vi "Grab and Bayer Decoding.vi"() -> ()   [LabVIEW 2011]
doc: "The Grab and Bayer Decoding VI acquires images continuously and displays the images in an image control using high-level acquisition VIs. This VI also demonstrates decoding bayer encoded patterns from the camera. A grab is appropriate for high-speed applications in which you need to process only one image at a time."
uses:
  <vilib>/vision/driver/NI_Vision_Acquisition_Software.lvlib
  resource/objmgr/imaqdx.rc
panel:
  in  "Camera Name":refnum<k21> caption="IMAQdx Session"
  in  "Bayer Parameters":T1 {"Blue Gain" scale=0.0..3.99; "Green Gain" scale=0.0..3.99; "Red Gain" scale=0.0..3.99; "Bayer Pattern" items=["None", "GB", "GR", "BG", "RG", "Use hardware value"]}
  out "Buffer Number":u32
  out "Image":T2(plugin-control)
  out "Frame Rate":dbl(knob) scale=0.0..100.0
  in  "Stop":bool
  # "Overview: Demonstrates how to modify the Bayer Parameters while acquiring a continuous acquisition.\nRequirements: Vision Acquisition Software, camera that outputs 8-bit or 16-bit Bayer images.\nInstructions: \n1. Select the Camera Name\n2. Run the VI\n3. Select the Bayer Pattern.\n4. Adjust the red, green, blue gains."
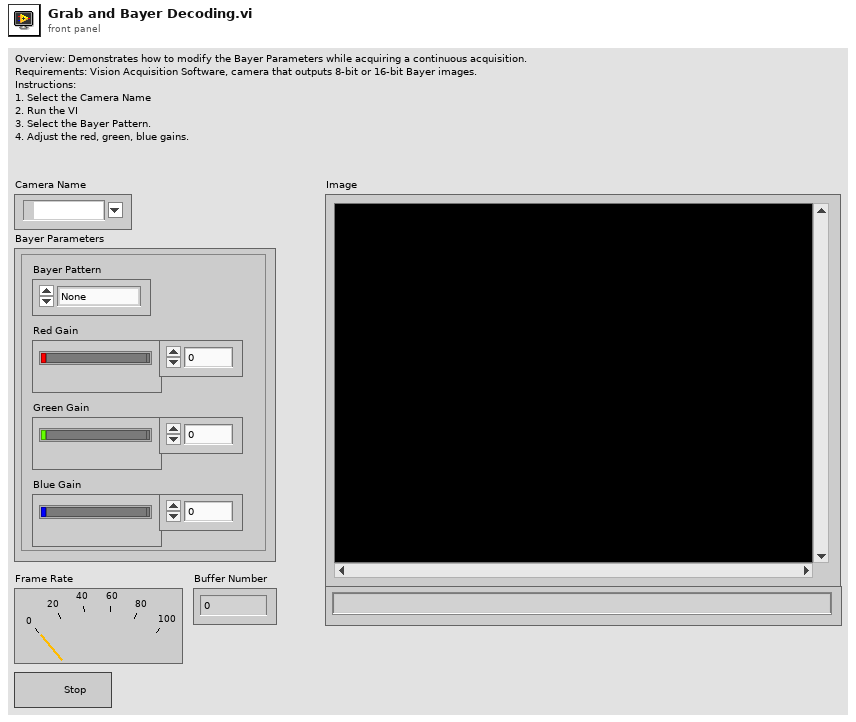
[diagram p1: front panel]
types:
  T1 = cluster{"Bayer Pattern":u32, "Red Gain":dbl, "Green Gain":dbl, "Blue Gain":dbl}
  T2 = typedef "IMAQ Image.ctl" = refnum<image>
  T3 = typedef "IMAQdx.ctl" = refnum<k21>
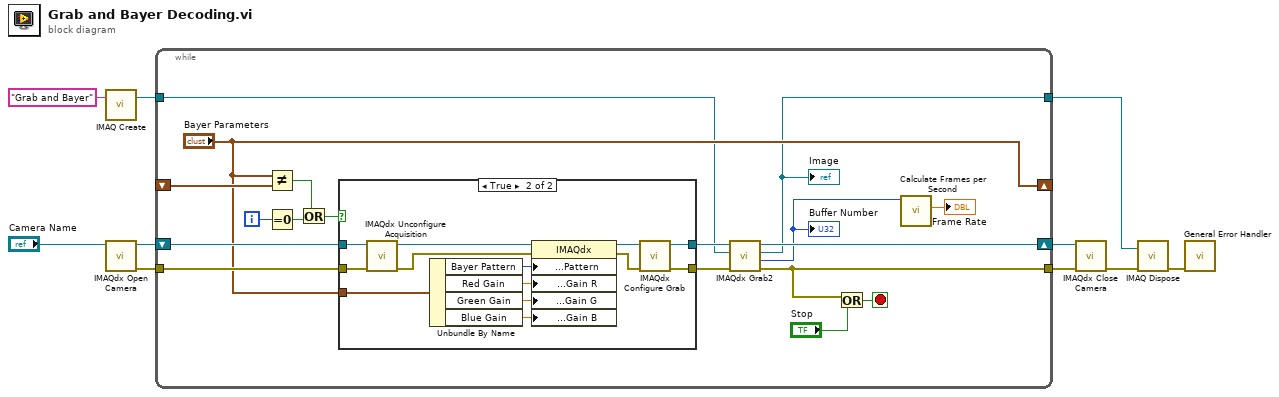
[diagram p0: block diagram]
diagram:
  n1 = call "IMAQ Create"("Image Name"="Grab and Bayer") -> ("New Image"=w10:T2)  [unwired: 3 in, 2 out]
  n2 = call <vilib>:"IMAQdx Open Camera.vi"("Session In"="Camera Name") -> ("error out"=w6:errorcluster, "Session Out"=w7:T3)  [unwired: 2 in, 7 out]
  n3 = while {
    tunnel: [w13] -> w8
    tunnel: w10 -> [w12]
    shift-right: ["Bayer Parameters"] -> _
    shift-left: _ -> [w21]
    tunnel: w6 -> [w22]
    shift-right: [w26] -> w9
    shift-left: w7 -> [w23]
    tunnel: [w11] -> w3
    i -> [w14]
    stop <- w28 stop-if-true
    n4 = Not Equal?(x="Bayer Parameters", y=w21) -> (x != y?=w16:bool)
    n5 = Equal To 0?(x=w14) -> (x = 0?=w20:bool)
    n6 = Or(x=w16, y=w20) -> (x .or. y?=w19:bool)
    n7 = case shown="True" w19 {
      tunnel: [w29 w43] -> w25
      tunnel: [w30 w42] -> w24
      tunnel: w23 -> [w30 w41]
      tunnel: w22 -> [w29 w39]
      tunnel: "Bayer Parameters" -> [_ w35]
      frame False {
      }
      frame True {
        n8 = call <vilib>:"IMAQdx Unconfigure Acquisition.vi"("error in"=w39, "Session In"=w41) -> ("error out"=w36:errorcluster, "Session Out"=w40:T3)  [unwired: 8 out]
        n9 = Unbundle By Name(w35) -> ("Bayer Pattern"=w34:u32, "Red Gain"=w33:dbl, "Green Gain"=w32:dbl, "Blue Gain"=w31:dbl)
        n10 = property class="IMAQdx"(reference=w40, error in=w36, "Acquisition Attributes:Bayer:Pattern"=w34, "Acquisition Attributes:Bayer:Gain R"=w33, "Acquisition Attributes:Bayer:Gain G"=w32, "Acquisition Attributes:Bayer:Gain B"=w31) -> (reference out=w38:T3, error out=w37:errorcluster)
        n11 = call <vilib>:"IMAQdx Configure Grab.vi"("error in"=w37, "Session In"=w38) -> ("error out"=w43:errorcluster, "Session Out"=w42:T3)  [unwired: 8 out]
      }
    }
    n12 = call <vilib>:"IMAQdx Grab2.vi"("error in"=w25, "Image In"=w12, "Session In"=w24) -> ("error out"=w13:errorcluster, "Buffer Number Out"=w17:u32, "Image Out"=w11:T2, "Session Out"=w26:T3)  [unwired: 5 in]
    "Image" <- w11
    "Buffer Number" <- w17
    n13 = Or(x=w13, y="Stop") -> (x .or. y?=w28:bool)
    n14 = call <vilib>:"Calculate Frames per Second.vi"("Buffer Number"=w17) -> ("Processed Frames/s"=→"Frame Rate":dbl)  [unwired: 8 in, 2 out]
  }
  n15 = call <vilib>:"IMAQdx Close Camera.vi"("error in"=w8, "Session In"=w9) -> ("error out"=w5:errorcluster)  [unwired: 9 out]
  n16 = call "IMAQ Dispose"("Image"=w3, "error in (no error)"=w5) -> ("error out"=w4:errorcluster)  [unwired: 4 in]
  n17 = call <vilib>:"General Error Handler.vi"("error in (no error)"=w4) -> ()  [unwired: 1 in, 14 out]
